vi "TestExec.Set Child Application Window State.vi"(1 "This VI":refnum<vi>) -> (0 "TE Running":bool)   [LabVIEW 2018]
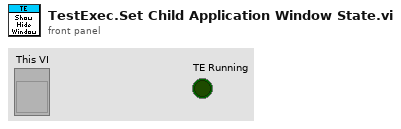
[diagram p1: front panel]
types:
  T1 = enum32{"invalid app kind", "Development System", "Run Time System", "Student Edition", "Embedded LabVIEW", "Evaluation", "Custom"}
  T2 = enum32{"Invalid", "Standard", "Closed", "Hidden", "Minimized", "Maximized"}
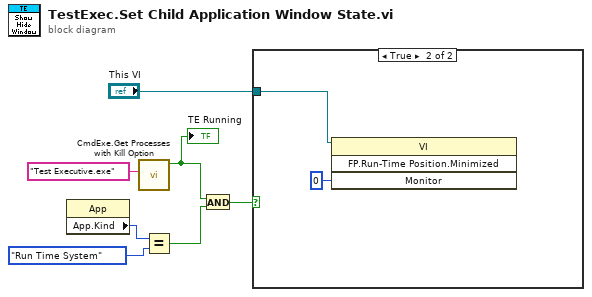
[diagram p0: block diagram]
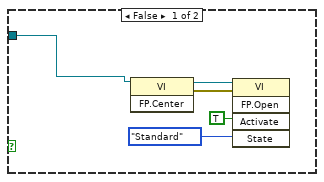
[diagram p2: hidden frame]
diagram:
  n1 = property class="App"() -> ("App.Kind"=w5:T1)  [unwired: 2 in, 2 out]
  n2 = call "CmdExe.Get Processes with Kill Option.vi"("Process Name"="Test Executive.exe") -> ("Is Running"=w1:bool)  [unwired: 7 in, 3 out]
  "TE Running" <- w1
  n3 = Equal?(x=w5, y=T1."Run Time System" ("Application:Kind")) -> (x = y?=w3:bool)
  n4 = And(x=w1, y=w3) -> (x .and. y?=w2:bool)
  n5 = case shown="True" w2 {
    tunnel: "This VI" -> [w8 w14]
    frame False {
      n6 = invoke class="VI" method="FP.Center"(reference=w8) -> (reference out=w11:refnum<vi>, error out=w12:errorcluster)  [unwired: 2 in, 1 out]
      n7 = invoke class="VI" method="FP.Open"(reference=w11, error in=w12, "Activate"=TRUE ("Activate?"), "State"=T2."Standard") -> ()  [unwired: 1 in, 5 out]
    }
    frame True {
      n8 = invoke class="VI" method="FP.Run-Time Position.Minimized"(reference=w14, "Monitor"=i16 0) -> ()  [unwired: 2 in, 4 out]
    }
  }
